vi "FTW-File-RebaseFilepath.vi"(0 "Original Path":path, 5 "Base Path":path, 7 "New Base Path":path) -> (4 "New Path":path, 6 "Original under Base?":bool)   [LabVIEW 2012]
uses:
  FTW-File-ValidateFilepath.vi
panel:
  # "Inputs"
  # "Outputs"
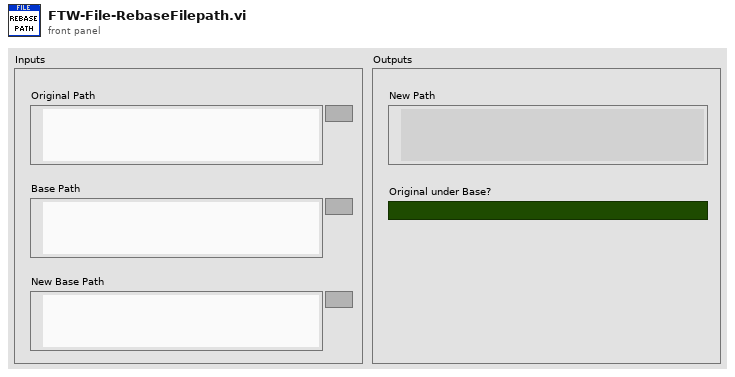
[diagram p1: front panel]
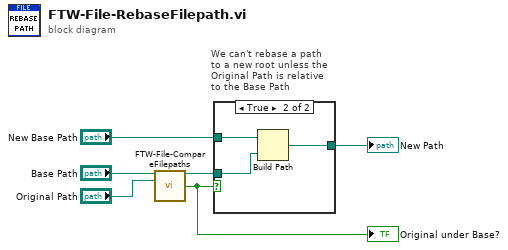
[diagram p0: block diagram]
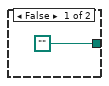
[diagram p2: hidden frame]
diagram:
  n1 = call "FTW-File-CompareFilepaths.vi"("Base Path"="Base Path", "Path to Compare"="Original Path") -> ("Relative Path from Base"=w2:path, "Path relative to Base?"=w1:bool)  [unwired: 11 in, 1 out]
  "Original under Base?" <- w1
  n2 = case "We can't rebase a path\nto a new root unless the\nOriginal Path is relative\nto the Base Path" shown="True" w1 {
    tunnel: "New Base Path" -> [_ w10]
    tunnel: [path "" w9] -> w5
    tunnel: w2 -> [_ w8]
    frame False {
    }
    frame True {
      n3 = Build Path(base path=w10, name or relative path=w8) -> (appended path=w9:path)
    }
  }
  "New Path" <- w5
